vi "Configure Digital Clock.vi"(0 "VISA resource name":refnum<visa-resource-name>, 1 "Clock Polarity (0: Positive)":u16(ring) items=["Positive", "Negative"], 2 "Clocks Per Sample (1)":u16(ring)=1 items=["1"=1, "2"=2, "4"=4], 5 "Clock Source (0: Internal)":u16(ring) items=["Internal", "External", "Device"], 7 "Clock Rate (100 MHz)":dbl=100000000.0, 9 "Clock Phase (0 deg)":dbl, 11 "error in (no error)":errorcluster, 12 "Reference Frequency (10 MHz)":dbl=10000000.0, 13 "Clock Skew (0 s)":dbl) -> (4 "VISA resource name out":refnum<visa-resource-name>, 15 "error out":errorcluster)   [LabVIEW 2018, in "Agilent PSG MXG Series.lvlib"]
doc: "Configures the clock signal.\n\n<B>Notes:</B>\n(1) This VI is valid in E8267D that installs <B>Option 601</B> or <B>Option 602</B> (Internal baseband generator), and <B>Option 003</B> (PSG digital output connectivity with N5102A) or <B>Option 004</B> (PSG digital input connectivity with N5102A).\n(2) This VI is valid in N5172B/82B that with <B> Option 003</B> or <B>Option 004</B> or <B>both</B>."
uses:
  Agilent PSG MXG Series.lvlib
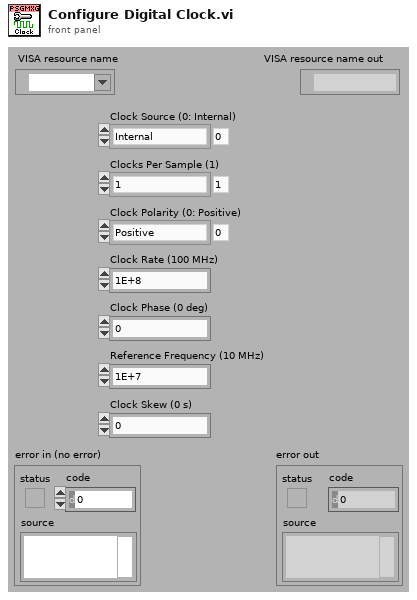
[diagram p1: front panel]
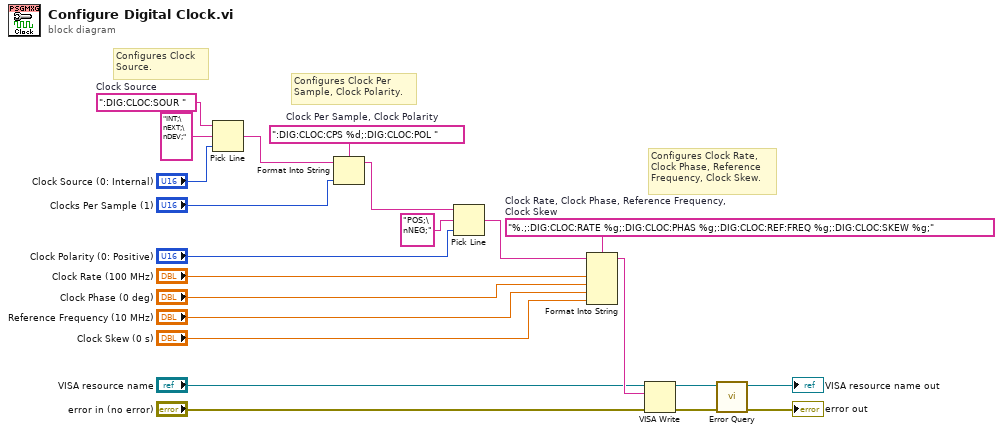
[diagram p0: block diagram]
diagram:
  w12 = "%.;:DIG:CLOC:RATE %g;:DIG:CLOC:PHAS %g;:DIG:CLOC:REF:FREQ %g;:DIG:CLOC:SKEW %g;"  # Clock Rate, Clock Phase, Reference Frequency, Clock Skew
  w18 = ":DIG:CLOC:CPS %d;:DIG:CLOC:POL "  # Clock Per Sample, Clock Polarity
  w22 = ":DIG:CLOC:SOUR "  # Clock Source
  # "Configures Clock Rate,\nClock Phase, Reference\nFrequency, Clock Skew."
  # "Configures Clock Per\nSample, Clock Polarity."
  # "Configures Clock\nSource."
  n1 = Pick Line(string ("")=w22, multi-line string="INT;\nEXT;\nDEV;", line index="Clock Source (0: Internal)") -> (output string=w19:string)
  n2 = Format Into String(format string=w18, initial string=w19, "Clocks Per Sample (1)") -> (resulting string=w16:string)  [unwired: 1 in, 1 out]
  n3 = Pick Line(string ("")=w16, multi-line string="POS;\nNEG;", line index="Clock Polarity (0: Positive)") -> (output string=w13:string)
  n4 = Format Into String(format string=w12, initial string=w13, "Clock Rate (100 MHz)", "Clock Phase (0 deg)", "Reference Frequency (10 MHz)", "Clock Skew (0 s)") -> (resulting string=w5:string)  [unwired: 1 in, 1 out]
  n5 = VISA Write(VISA resource name="VISA resource name", write buffer=w5, error in (no error)="error in (no error)") -> (VISA resource name out=w7:refnum<visa-resource-name>, error out=w6:errorcluster)  [unwired: 1 out]
  n6 = call "Error Query.vi"("error in (no error)"=w6, "VISA resource name"=w7) -> ("error out"=→"error out":errorcluster, "VISA resource name out"=→"VISA resource name out":refnum<visa-resource-name>)  [unwired: 8 out]
